vi "Write Enum Reference.vi"(8 "error in (no error)":errorcluster, 10 "Enum Reference":refnum<vi>, 11 "List Box Enum Column in":refnum<class "List Box Enum Column.lvclass">) -> (0 "error out":errorcluster, 3 "List Box Enum Column out":refnum<class "List Box Enum Column.lvclass">)   [LabVIEW 2013, in "Table Manager.lvlib" / "List Box Enum Column.lvclass"]
uses:
  List Box Enum Column.lvclass
  <vilib>/NI/Tag Bus/tag/Data Type.ctl
  List Box Enum Column.lvclass/List Box Enum Column.ctl
  <vilib>/NI/Tag Bus/tag/tag descriptor.lvclass
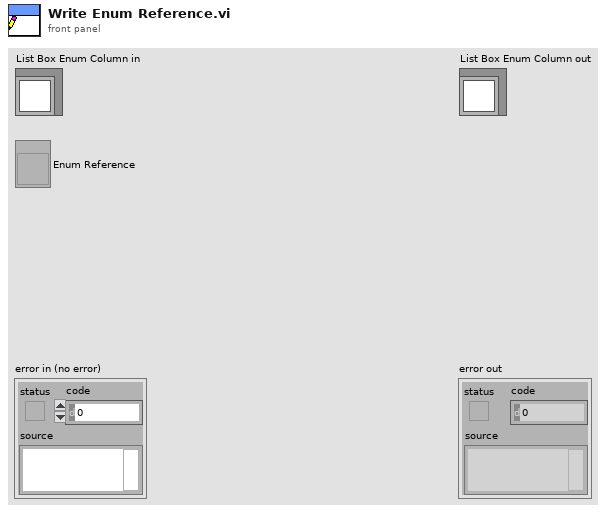
[diagram p1: front panel]
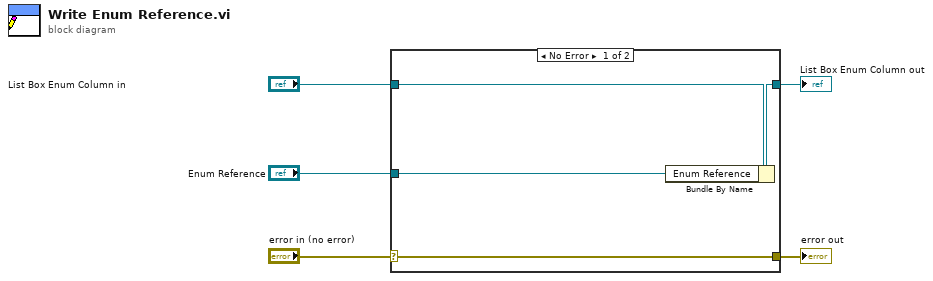
[diagram p0: block diagram]
diagram:
  n1 = case shown="No Error" "error in (no error)" {
    selector: "error in (no error)" -> [w9 w10]
    tunnel: [w9 w10] -> w4
    tunnel: [w7 w11] -> w2
    tunnel: "List Box Enum Column in" -> [w8 w11]
    tunnel: "Enum Reference" -> [w6 _]
    frame No Error {
      n2 = Bundle By Name(cluster=w8, "Enum Reference"=w6) -> (w7:refnum<class "List Box Enum Column.lvclass">)
    }
    frame Error {
    }
  }
  "error out" <- w4
  "List Box Enum Column out" <- w2
